vi "PH_PP_CurrentMeas.evt call Select MA BO.vi"(0 "i ref in":refnum<vi>, 2 "Instance name":string, 3 "Select MA BO":bool, 5 "error in (no error)":errorcluster) -> (14 "i ref out":refnum<vi>, 19 "error out":errorcluster)   [LabVIEW 2014, in "PH_PP_CurrentMeas.lvlib"]
doc: "This VI calls an event by a simple call."
uses:
  PH_PP_CurrentMeas.lvlib
  CSCore/CSSystem/CoreLib/CoreLib.short 2 byte array.vi
  CSCore/CSSystem/CoreLib/CoreLib.lvlib
  CSCore/BaseProcess/BaseProcess.lvlib
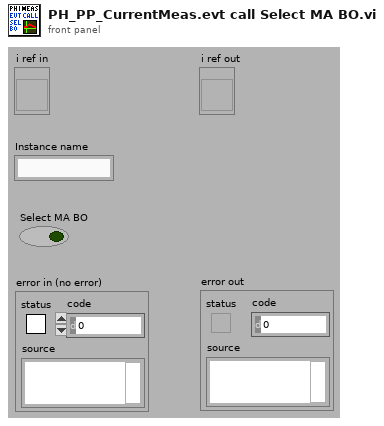
[diagram p1: front panel]
types:
  T1 = typedef "CoreDefs.rawDataType.ctl" = i8[]
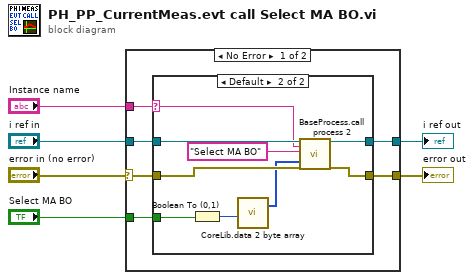
[diagram p0: block diagram]
diagram:
  n1 = case shown="No Error" "error in (no error)" {
    selector: "error in (no error)" -> [w8 w24]
    tunnel: "Select MA BO" -> [w12 _]
    tunnel: "Instance name" -> [w7 _]
    tunnel: "i ref in" -> [w11 w25]
    tunnel: [w10 w25] -> w2
    tunnel: [w9 w24] -> w1
    frame No Error {
      n2 = case shown="Default" w7 {
        selector: w7 -> [_ w15]
        tunnel: w12 -> [_ w18]
        tunnel: w8 -> [w13 w22]
        tunnel: w11 -> [w14 w21]
        tunnel: [w14 w20] -> w10
        tunnel: [w13 w19] -> w9
        frame "N/A" {
        }
        frame Default {
          n3 = Boolean To (0,1)(Boolean=w18) -> (0, 1=w17:i16)
          n4 = call-poly "CoreLib.data 2 byte array.vi"("i16"=w17) -> ("byteArray out"=w16:T1)  [unwired: 18 in]
          n5 = call "BaseProcess.call process 2.vi"("i ref in"=w21, "Object"=w15, "Selector"="Select MA BO", "Data"=w16, "error in (no error)"=w22) -> ("i ref out"=w20:refnum<vi>, "error out"=w19:errorcluster)  [unwired: 13 in]
        }
      }
    }
    frame Error {
    }
  }
  "error out" <- w1
  "i ref out" <- w2
